vi "music-learner-fpga.vi"() -> ()   [LabVIEW 2015]
uses:
  <vilib>/rvi/Emulation/niFpgaGetClockAttributes.vi
  <vilib>/rvi/Emulation/niFpgaSctlEmulationGetInTimedLoop.vi
  <vilib>/rvi/Emulation/niFpgaEmulationReportErrorSimple.vi
  <vilib>/rvi/Emulation/niFpgaCriticalErrorInLSC.vi
panel:
  out "output 3":i16
  out "output 2":i16
  out "output 1":i16
  in  "w213":fxp<+/-,64,32>
  in  "w212":fxp<+/-,64,32>
  in  "w211":fxp<+/-,64,32>
  in  "w223":fxp<+/-,64,32>
  in  "w222":fxp<+/-,64,32>
  in  "w221":fxp<+/-,64,32>
  in  "w233":fxp<+/-,64,32>
  in  "w232":fxp<+/-,64,32>
  in  "w231":fxp<+/-,64,32>
  in  "w113":fxp<+/-,64,32>
  in  "w112":fxp<+/-,64,32>
  in  "w111":fxp<+/-,64,32>
  in  "w123":fxp<+/-,64,32>
  in  "w122":fxp<+/-,64,32>
  in  "w121":fxp<+/-,64,32>
  in  "w133":fxp<+/-,64,32>
  in  "w132":fxp<+/-,64,32>
  in  "w131":fxp<+/-,64,32>
  in  "stop":bool
  in  "input 3":fxp<+/-,64,32>
  in  "input 2":fxp<+/-,64,32>
  in  "input 1":fxp<+/-,64,32>
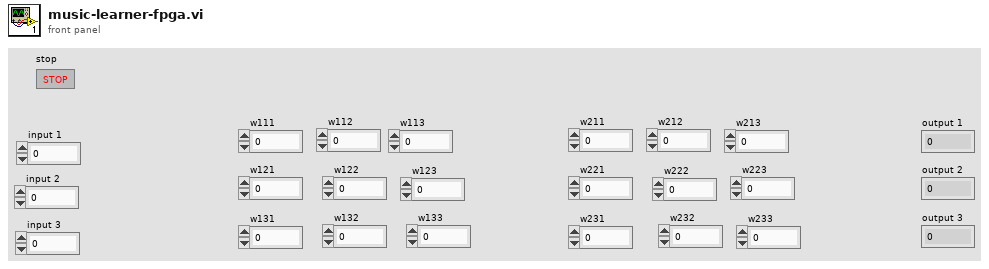
[diagram p1: front panel]
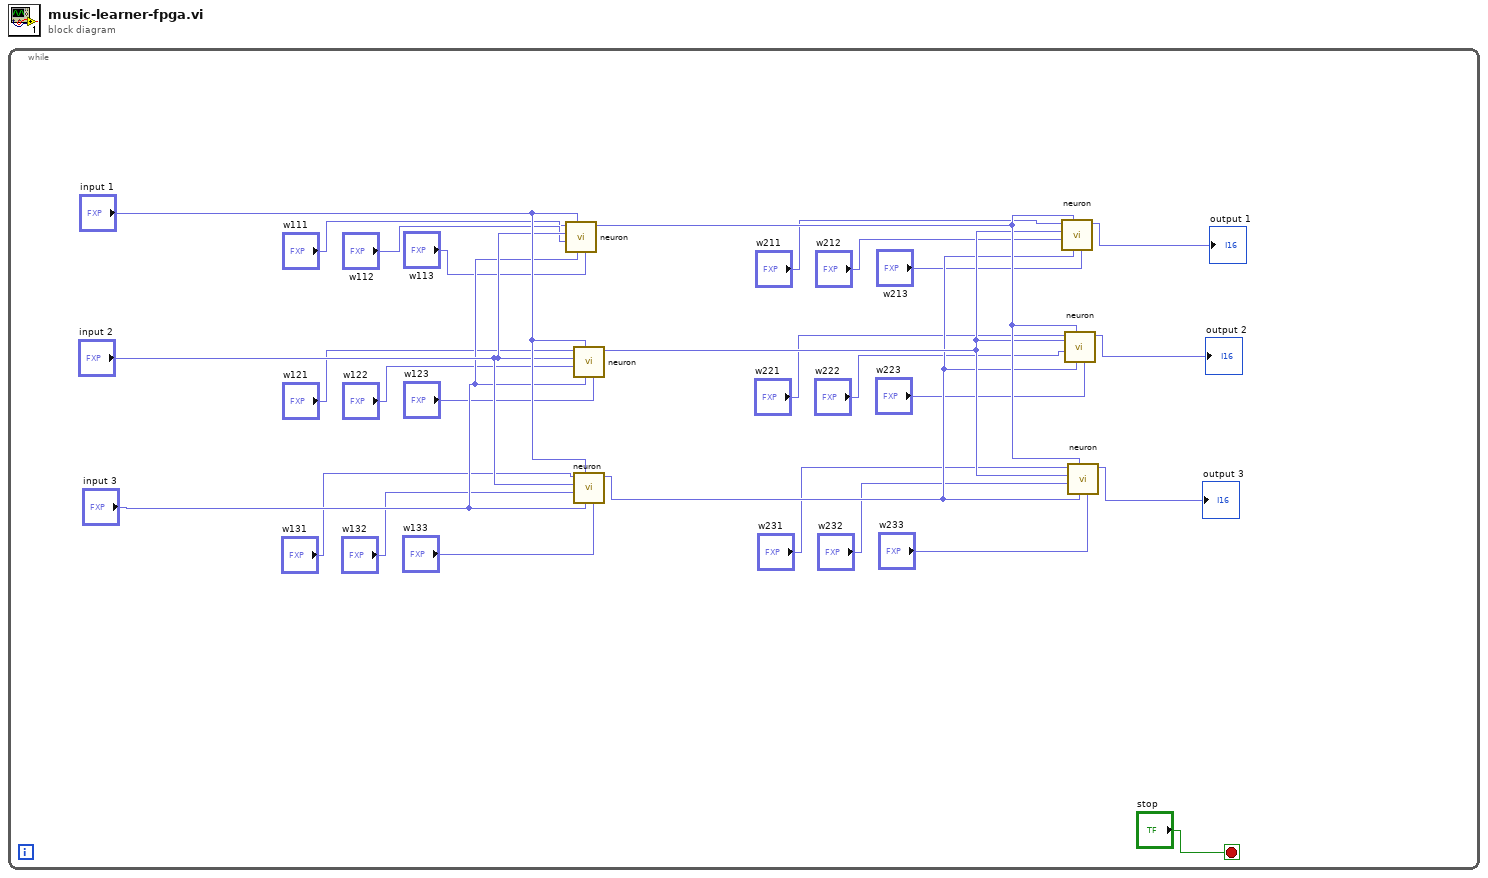
[diagram p0: block diagram]
diagram:
  n1 = while {
    stop <- "stop" stop-if-true
    n2 = call "neuron.vi"("weight 3"="w113", "input 3"="input 3", "input 1"="input 1", "weight 2"="w112", "input 2"="input 2", "weight 1"="w111") -> ("activation"=w27:fxp<+/-,64,32>)  [unwired: 5 in]
    n3 = call "neuron.vi"("weight 3"="w123", "input 3"="input 3", "input 1"="input 1", "weight 2"="w122", "input 2"="input 2", "weight 1"="w121") -> ("activation"=w26:fxp<+/-,64,32>)  [unwired: 5 in]
    n4 = call "neuron.vi"("weight 3"="w133", "input 3"="input 3", "input 1"="input 1", "weight 2"="w132", "input 2"="input 2", "weight 1"="w131") -> ("activation"=w25:fxp<+/-,64,32>)  [unwired: 5 in]
    n5 = call "neuron.vi"("weight 3"="w213", "input 3"=w25, "input 1"=w27, "weight 2"="w212", "input 2"=w26, "weight 1"="w211") -> ("activation"=→"output 1":fxp<+/-,64,32>)  [unwired: 5 in]
    n6 = call "neuron.vi"("weight 3"="w223", "input 3"=w25, "input 1"=w27, "weight 2"="w222", "input 2"=w26, "weight 1"="w221") -> ("activation"=→"output 2":fxp<+/-,64,32>)  [unwired: 5 in]
    n7 = call "neuron.vi"("weight 3"="w233", "input 3"=w25, "input 1"=w27, "weight 2"="w232", "input 2"=w26, "weight 1"="w231") -> ("activation"=→"output 3":fxp<+/-,64,32>)  [unwired: 5 in]
  }
